vi "finishPreparePassInGame1.vi"(7 "OffensiveTeam in":refnum<class "Ally.lvclass">, 8 "error in (no error)":errorcluster, 9 "command_interpreted":T1, 10 "Game in":refnum<class "Game.lvclass">, 11 "PreparePassInGame1 in":refnum<class "PreparePassInGame1.lvclass">) -> (0 "error out":errorcluster, 1 "finished?":bool, 2 "OffensiveTeam out":refnum<class "Ally.lvclass">, 3 "PreparePassInGame1 out":refnum<class "PreparePassInGame1.lvclass">)   [LabVIEW 2020, in "PreparePassInGame1.lvclass"]
uses:
  PreparePassInGame1.lvclass
  Referee_class/command_interpreted.ctl
  Game_class/Game.lvclass
  Ally_class/Ally.lvclass
  C:/Users/anton/Desktop/RoboIME/IC/SSL_AI/Team_class/Team.lvclass
  Robot_class/roles.ctl
  Utilities_class/Utilities.lvclass
  Game_class/Game.lvclass/Game.ctl
  Referee_class/Referee.lvclass/Referee.ctl
  Events_class/Events.lvclass/Events.ctl
  Object_class/Object.lvclass/Object.ctl
  Team_class/Team.lvclass/Team.ctl
  Team_class/OffensivePlay.ctl
  Robot_class/Robot.lvclass/Robot.ctl
  Robot_class/Read dest_x_kick.vi
  Robot_class/Read dest_y_kick.vi
  Object_class/Read x.vi
  Object_class/Read y.vi
  Team_class/Read RobotRef.vi
  Game_class/Read Referee.vi
  Game_class/Read EventsRef.vi
  Game_class/Read Utilities.lvclass.vi
  Game_class/Read BallRef.vi
  Game_class/Read FieldRef.vi
  Game_class/Read EnemyRef.vi
  Events_class/Read id_touch.vi
  Events_class/Read touch.vi
  Events_class/Read enemy_ball_possesion.vi
  Events_class/Read ball_out.vi
  Referee_class/Read command_interpreted.vi
  Ball_class/Ball.lvclass
  C:/Users/anton/Desktop/RoboIME/IC/SSL_AI/Object_class/Object.lvclass
  Robot_class/Robot.lvclass
  Referee_class/Referee.lvclass
  Events_class/Events.lvclass
  Field_class/Field.lvclass
  Enemy_class/Enemy.lvclass
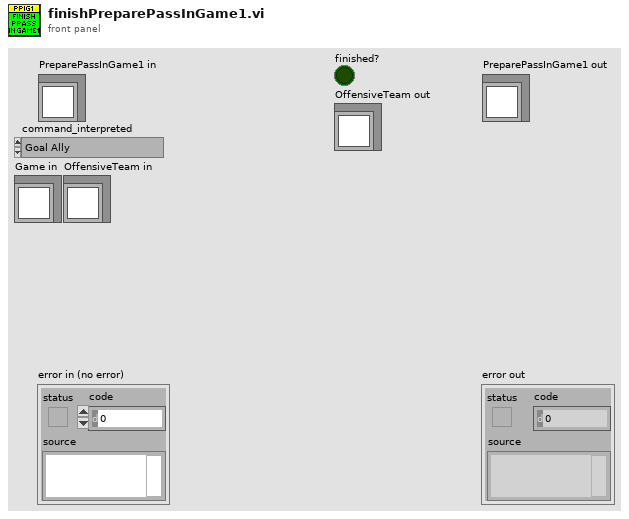
[diagram p1: front panel]
types:
  T1 = typedef "command_interpreted.ctl" = enum16{"Goal Ally", "Goal Enemy", "Ball Placement Enemy", "Ball Placement Ally", "Normal Half Time", "Extra Time  Break", "Extra Half Time", "None", "Post Game", "PKA Normal Start", "Prepare Kickoff Ally", "PKE Normal Start", "Prepare Kickoff Enemy", "Force Start", "Halt", "Timeout", "Prepare Penalty Ally", "Prepare Penalty Enemy", "PPA NormalStart", "PPE Normal Start", "Indirect Free Ally", "Direct Free Enemy", "Direct Free Ally", "Indirect Free Enemy", "Stop"}
  T2 = typedef "roles.ctl" = enum16{"SimpleBallPlacement", "BallPlacementAllyPasser", "BallPlacementAllyReceiver", "BallPlacementEnemy", "5Robots5th", "PassBestReceiver", "5Robots4th", "5Robots3rd", "5Robots2nd", "5Robots1st", "PassBestRobot", "WaitPass", "ABCThirdKicker", "ABCFirstKicker", "ABCSecondKicker", "Tabler", "TableFinalizer", "PrepareRollToPassRoller", "PrepareRollToPassReceiver", "SimplePassRoll", "SimplePassRollReceiver", "PenaltyDefense", "PreparePassReceiver 2", "PreparePassReceiver 1", "PassObserver", "Timeout", "Goto", "ZigZag", "None", "BallOutOfField", "DefenderArea", "Duelist", "AttackerStop", "FollowAttacker", "KeeperRole", "KickPenalty", "AttackerAimGoal", "AttackerBlock", "Marker", "Halt", "Shoot", "PassKicker", "PassReceiver", "TestRole", "PenaltyAttacker"}
  T3 = typedef "OffensivePlay.ctl" = enum16{"5RobotsPassGamePlay", "5PreparePassGame", "5RobotsKeeperGame", "KeeperPassToStriker", "5RobotsNormalGamePlay", "PrepareKeeperPass", "ACBPass", "ABCPass", "PrepareTriplePass", "TableWithStriker", "TableWith2ndStrikerPlay", "PrepareDoublePass", "PrepareRollToPass", "SimplePass", "PreparePass", "PassToStriker", "BallOutOfField", "PassTo2ndStriker", "StopOffensive", "Prepare Penalty Enemy", "EnemyPossessionAtEnemyField", "EnemyPossesionAtOurField", "TestPlay", "PreparePenaltyAlly", "KickPenaltyAlly", "PrepareKickoffAlly", "PrepareKickoffEnemy", "IndirectEnemy", "DirectEnemy", "PreparePassInGame1", "NormalGame", "DirectKick", "Pass", "Halt", "Timeout", "PassPlay", "PenaltyEnemy"}
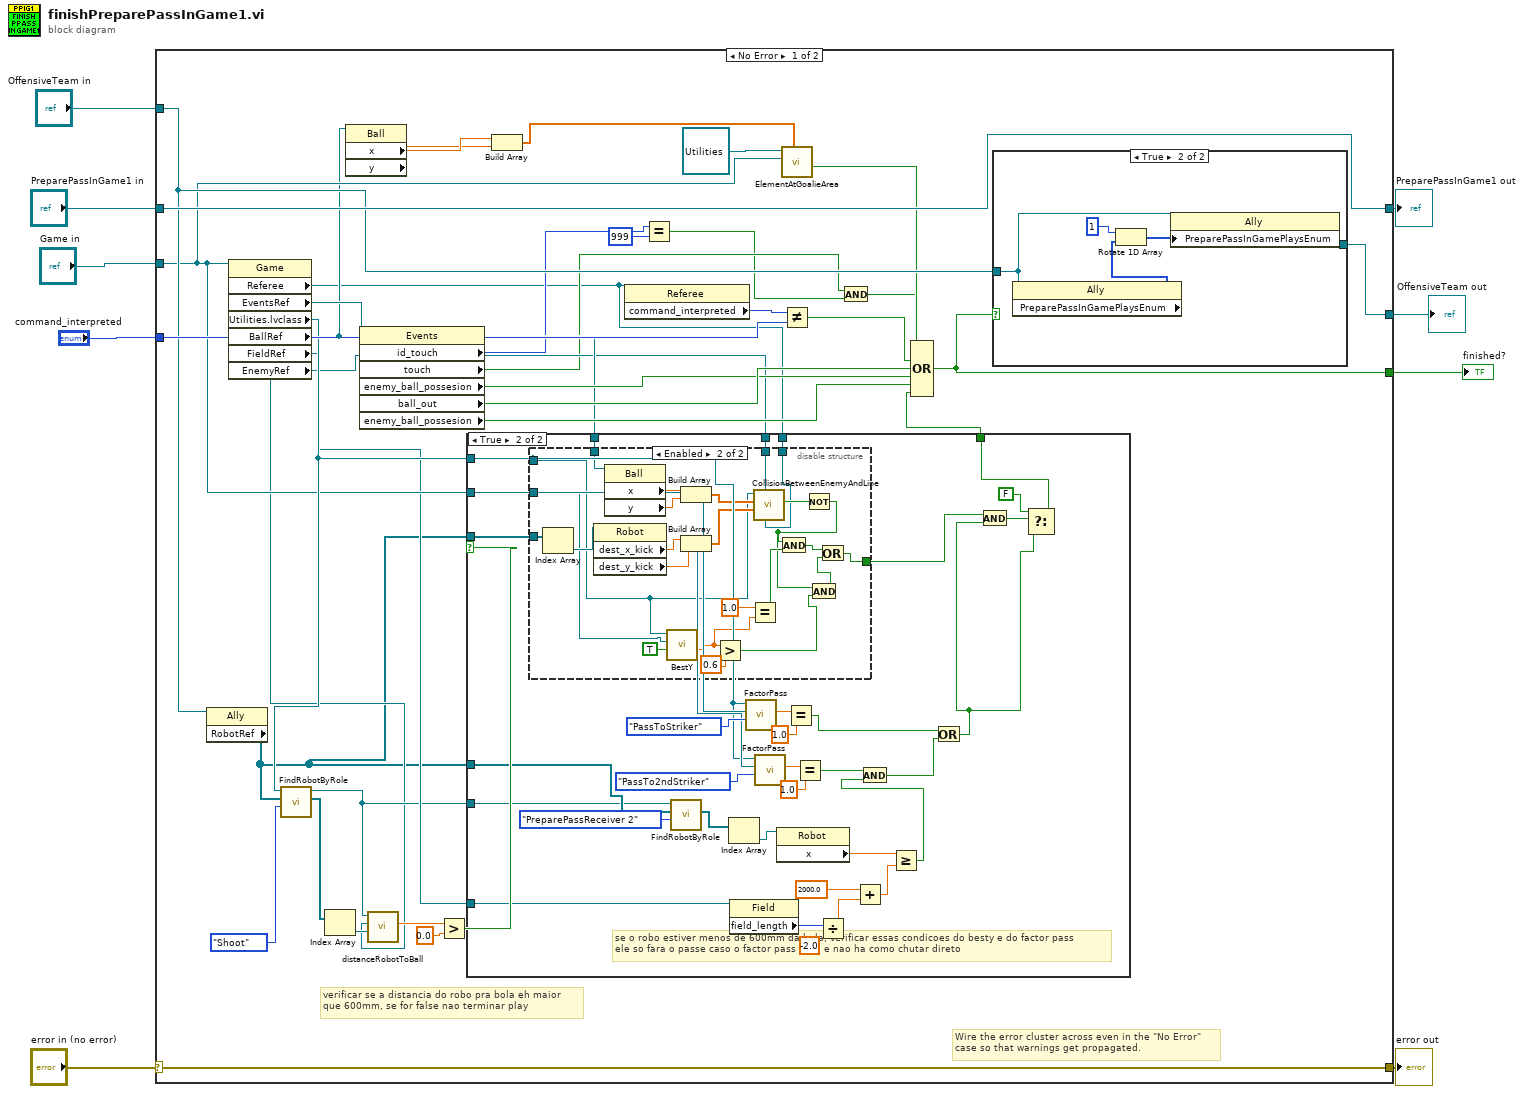
[diagram p0: block diagram]
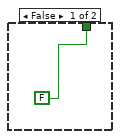
[diagram p2: hidden frame]
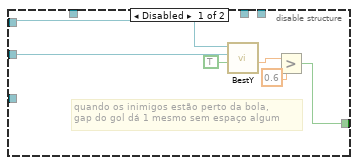
[diagram p3: hidden frame]
diagram:
  n1 = case shown="No Error" "error in (no error)" {
    selector: "error in (no error)" -> [w46 w118]
    tunnel: [w46 w118] -> w8
    tunnel: [w36 w117] -> w6
    tunnel: "PreparePassInGame1 in" -> [w36 w117]
    tunnel: "command_interpreted" -> [w39 _]
    tunnel: [w38 _] -> w1
    tunnel: "Game in" -> [w22 _]
    tunnel: "OffensiveTeam in" -> [w33 _]
    tunnel: [w37 _] -> w2
    frame No Error {
      # "verificar se a distancia do robo pra bola eh maior \nque 600mm, se for false nao terminar play"
      # "Wire the error cluster across even in the \"No Error\"\ncase so that warnings get propagated."
      n2 = property class="Ally"(reference=w33) -> ("RobotRef"=w17:refnum<class "Robot.lvclass">[])  [unwired: 1 in, 2 out]
      n3 = property class="Game"(reference=w22) -> ("Referee"=w10:refnum<class "Referee.lvclass">, "EventsRef"=w41:refnum<class "Events.lvclass">, "Utilities.lvclass"=w35:refnum<class "Utilities.lvclass">, "BallRef"=w18:refnum<class "Ball.lvclass">, "FieldRef"=w20:refnum<class "Field.lvclass">, "EnemyRef"=w16:refnum<class "Enemy.lvclass">)  [unwired: 1 in, 2 out]
      n4 = call "FindRobotByRole.vi"("role"=roles."Shoot", "RobotRef"=w17, "Utilities in"=w35) -> ("Robots"=w32:refnum<class "Robot.lvclass">[], "Utilities out"=w19:refnum<class "Utilities.lvclass">)  [unwired: 6 in, 1 out]
      n5 = Index Array(array=w32) -> (element=w31:refnum<class "Robot.lvclass">)  [unwired: 1 in]
      n6 = property class="Ball"(reference=w18) -> ("x"=w25:dbl, "y"=w24:dbl)  [unwired: 1 in, 2 out]
      n7 = property class="Events"(reference=w41) -> ("id_touch"=w14:i32, "touch"=w15:bool, "enemy_ball_possesion"=w43:bool, "ball_out"=w44:bool, "enemy_ball_possesion"=w45:bool)  [unwired: 1 in, 2 out]
      n8 = call "distanceRobotToBall.vi"("Robot"=w31, "Ball"=w18, "Utilities in"=w19) -> ("Distance Robot To Ball"=w30:dbl)  [unwired: 6 in, 2 out]
      n9 = Greater?(x=w30, y=0.0) -> (0:w27:bool)
      n10 = case shown="True" w27 {
        tunnel: w22 -> [_ w70]
        tunnel: w35 -> [_ w67]
        tunnel: [FALSE w74] -> w28
        tunnel: w17 -> [_ w64]
        tunnel: w20 -> [_ w53]
        tunnel: w19 -> [_ w52]
        tunnel: w18 -> [_ w51]
        tunnel: w17 -> [_ w50]
        tunnel: w16 -> [_ w49]
        tunnel: w10 -> [_ w48]
        frame False {
        }
        frame True {
          # "se o robo estiver menos de 600mm da bola, verificar essas condicoes do besty e do factor pass\nele so fara o passe caso o factor pass for 1 e nao ha como chutar direto"
          n11 = disable-structure shown="Enabled" {
            disable-tunnel: [w83 w93] -> w77
            disable-tunnel: w70 -> [w82 w96]
            disable-tunnel: w67 -> [w81 w97]
            disable-tunnel: w51 -> [_ w110]
            disable-tunnel: w50 -> [_ w106]
            disable-tunnel: w49 -> [_ w101]
            disable-tunnel: w48 -> [_ w87]
            frame Disabled {
              # "quando os inimigos estão perto da bola,\ngap do gol dá 1 mesmo sem espaço algum"
              n12 = call "BestY.vi"("Utilities in"=w81, "Game"=w82, "inimigos"=TRUE) -> ("Gap kick"=w85:dbl)  [unwired: 2 in, 4 out]
              n13 = Greater?(x=w85, y=0.6) -> (0:w83:bool)
            }
            frame Enabled {
              n14 = Index Array(array=w106) -> (element=w105:refnum<class "Robot.lvclass">)  [unwired: 1 in]
              n15 = property class="Robot"(reference=w105) -> ("dest_x_kick"=w104:dbl, "dest_y_kick"=w103:dbl)  [unwired: 1 in, 2 out]
              n16 = property class="Ball"(reference=w110) -> ("x"=w109:dbl, "y"=w108:dbl)  [unwired: 1 in, 2 out]
              n17 = call "BestY.vi"("Utilities in"=w97, "Game"=w96, "inimigos"=TRUE) -> ("Gap kick"=w95:dbl)  [unwired: 2 in, 4 out]
              n18 = Build Array(w109, w108) -> (w107:dbl[])
              n19 = Build Array(w104, w103) -> (w102:dbl[])
              n20 = Greater?(x=w95, y=0.6) -> (0:w90:bool)
              n21 = Equal?(x=1.0, y=w95) -> (x = y?=w91:bool)
              n22 = call-dynamic "CollisionBetweenEnemyAndLine.vi"("Referee"=w87, "EnemyRef"=w101, "P2"=w102, "P1"=w107, "Utilities in"=w97) -> ("collision ?"=w100:bool)  [unwired: 3 in, 3 out]
              n23 = Not(x=w100) -> (.not. x?=w89:bool)
              n24 = And(x=w89, y=w91) -> (x .and. y?=w92:bool)
              n25 = And(x=w89, y=w90) -> (x .and. y?=w88:bool)
              n26 = Or(x=w92, y=w88) -> (x .or. y?=w93:bool)
            }
          }
          n27 = call "FindRobotByRole.vi"("role"=roles."PreparePassReceiver 2", "RobotRef"=w64, "Utilities in"=w52) -> ("Robots"=w55:refnum<class "Robot.lvclass">[])  [unwired: 6 in, 2 out]
          n28 = Index Array(array=w55) -> (element=w62:refnum<class "Robot.lvclass">)  [unwired: 1 in]
          n29 = property class="Field"(reference=w53) -> ("field_length"=w60:i32)  [unwired: 1 in, 2 out]
          n30 = call-dynamic "FactorPass.vi"("OffensivePlay"=OffensivePlay."PassToStriker", "Game"=w70, "Utilities in"=w67) -> ("Critério de marcação Normalizado"=w79:dbl)  [unwired: 6 in, 2 out]
          n31 = call-dynamic "FactorPass.vi"("OffensivePlay"=OffensivePlay."PassTo2ndStriker", "Game"=w70, "Utilities in"=w67) -> ("Critério de marcação Normalizado"=w72:dbl)  [unwired: 6 in, 2 out]
          n32 = property class="Robot"(reference=w62) -> ("x"=w61:dbl)  [unwired: 1 in, 2 out]
          n33 = Equal?(x=w79, y=1.0) -> (x = y?=w69:bool)
          n34 = Equal?(x=w72, y=1.0) -> (x = y?=w65:bool)
          n35 = Divide(x=w60, y=-2.0) -> (x/y=w58:dbl)
          n36 = Add(x=2000.0, y=w58) -> (x+y=w57:dbl)
          n37 = Greater Or Equal?(x=w61, y=w57) -> (x >= y?=w54:bool)
          n38 = And(x=w65, y=w54) -> (x .and. y?=w66:bool)
          n39 = Or(x=w69, y=w66) -> (x .or. y?=w68:bool)
          n40 = And(x=w77, y=w68) -> (x .and. y?=w76:bool)
          n41 = Select(t=FALSE, s=w76, f=w68) -> (s? t:f=w74:bool)
        }
      }
      n42 = Build Array(w25, w24) -> (w23:dbl[])
      n43 = property class="Referee"(reference=w10) -> ("command_interpreted"=w40:T1)  [unwired: 1 in, 2 out]
      n44 = Equal?(x=w14, y=999) -> (x = y?=w12:bool)
      n45 = call "ElementAtGoalieArea.vi"("Elemento pos."=w23, "Game"=w22, "Utilities in"=refnum<class "Utilities.lvclass"> refnum) -> ("Element at our goalkeeper area ?"=w21:bool)  [unwired: 4 in, 4 out]
      n46 = Not Equal?(x=w40, y=w39) -> (x != y?=w42:bool)
      n47 = And(x=w15, y=w12) -> (x .and. y?=w11:bool)
      n48 = Compound Arithmetic op=OR(w11, w21, w42, w44, w43, w45, w28) -> (w38:bool)
      n49 = case shown="True" w38 {
        tunnel: [w111 w114] -> w37
        tunnel: w33 -> [w111 w113]
        frame False {
        }
        frame True {
          n50 = property class="Ally"(reference=w113) -> ("PreparePassInGamePlaysEnum"=w112:T3[])  [unwired: 1 in, 2 out]
          n51 = Rotate 1D Array(1:w112, 2:1 ("n")) -> (0:w115:T3[])
          n52 = property class="Ally"(reference=w113, "PreparePassInGamePlaysEnum"=w115) -> (reference out=w114:refnum<class "Ally.lvclass">)  [unwired: 1 in, 1 out]
        }
      }
    }
    frame Error {
    }
  }
  "error out" <- w8
  "PreparePassInGame1 out" <- w6
  "finished?" <- w1
  "OffensiveTeam out" <- w2
